vi "new_win.vi"(0 "Nota 3":string, 1 "Nota 2":string, 2 "Nota 01":string, 3 "File name":string, 4 "OK Button":bool) -> ()   [LabVIEW 2011]
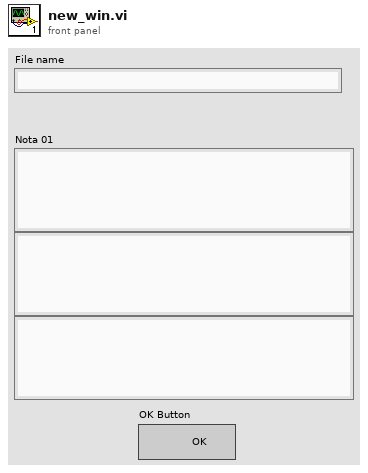
[diagram p1: front panel]
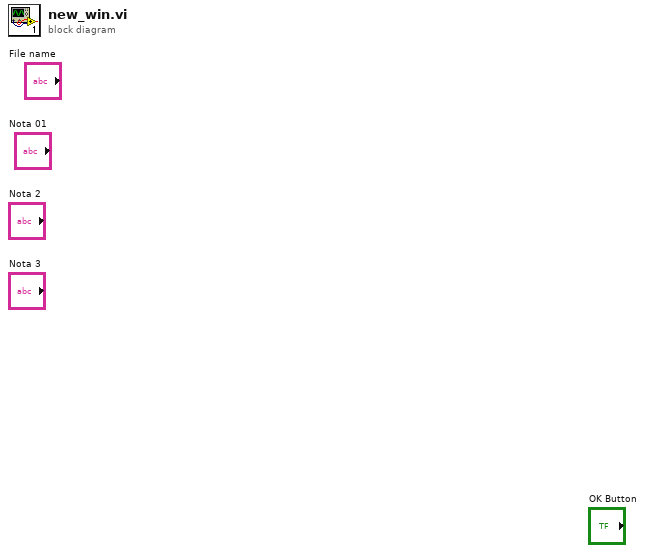
[diagram p0: block diagram]
diagram:
